vi "Set Version Number.vi"(8 "error in (no error)":errorcluster, 10 "Version number":T1, 11 "DSDIST in":refnum<class "NI_AB_API_DSDIST.lvclass">) -> (0 "error out":errorcluster, 3 "DSDIST out":refnum<class "NI_AB_API_DSDIST.lvclass">)   [LabVIEW 2020, in "NI_AB_API_DSDIST.lvclass"]
uses:
  <vilib>/AppBuilder/AB_API/DSDIST/NI_AB_API_DSDIST.lvclass
  <vilib>/AppBuilder/AB_API/common/AB_API Version Number.ctl
  <vilib>/AppBuilder/AB_API/SDIST/NI_AB_API_SDIST.lvclass
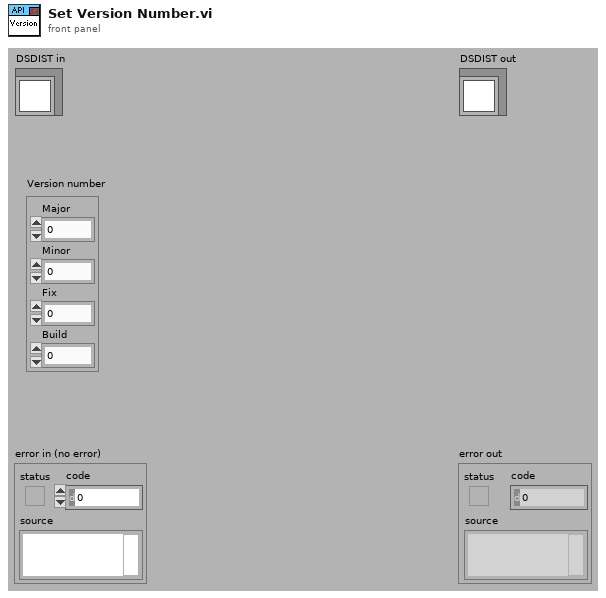
[diagram p1: front panel]
types:
  T1 = typedef "AB_API Version Number.ctl" = cluster{"Major":u16, "Minor":u16, "Fix":u16, "Build":u16}
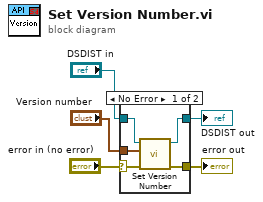
[diagram p0: block diagram]
diagram:
  n1 = case shown="No Error" "error in (no error)" {
    selector: "error in (no error)" -> [w6 w12]
    tunnel: [w7 w12] -> w4
    tunnel: [w9 w11] -> w2
    tunnel: "DSDIST in" -> [w10 w11]
    tunnel: "Version number" -> [w8 _]
    frame No Error {
      n2 = call-parent "Set Version Number.vi"("error in (no error)"=w6, "Version number"=w8, "SDIST in"=w10) -> ("error out"=w7:errorcluster, "SDIST out"=w9:refnum<class "NI_AB_API_DSDIST.lvclass">)  [unwired: 7 in]
    }
    frame Error {
    }
  }
  "error out" <- w4
  "DSDIST out" <- w2
